vi "enablePWM.vi"(0 "MotorControllerClass in":refnum<class "MotorControllerClass.lvclass">, 3 "error in (no error)":errorcluster) -> (7 "MotorControllerClass out":refnum<class "MotorControllerClass.lvclass">, 10 "error out":errorcluster)   [LabVIEW 2018, in "MotorControllerClass.lvclass"]
uses:
  BMS/MotorControllerClass.lvclass
  <vilib>/CANopenLib/CANOPEN.llb/CANopen Convert To Data [U16].vi
  <vilib>/CANopenLib/CANOPEN.llb/CANopen Convert To Data [I32].vi
  <vilib>/CANopenLib/CANOPEN.llb/CANopen Convert To Data [I16].vi
panel:
  in  "targetVelocity":i32
  in  "targetTorque":i16
  out "interface object out":refnum<k20>
  in  "interface object in":refnum<k20>
  in  "CANopen data in":u8[](array[numeric])=[0, 0, 0, 0, 0, 0, 0, 0] format="%.0x"
  in  "PDOChannel":u8(ring) items=["PDO 1", "PDO 2", "PDO 3", "PDO 4"]
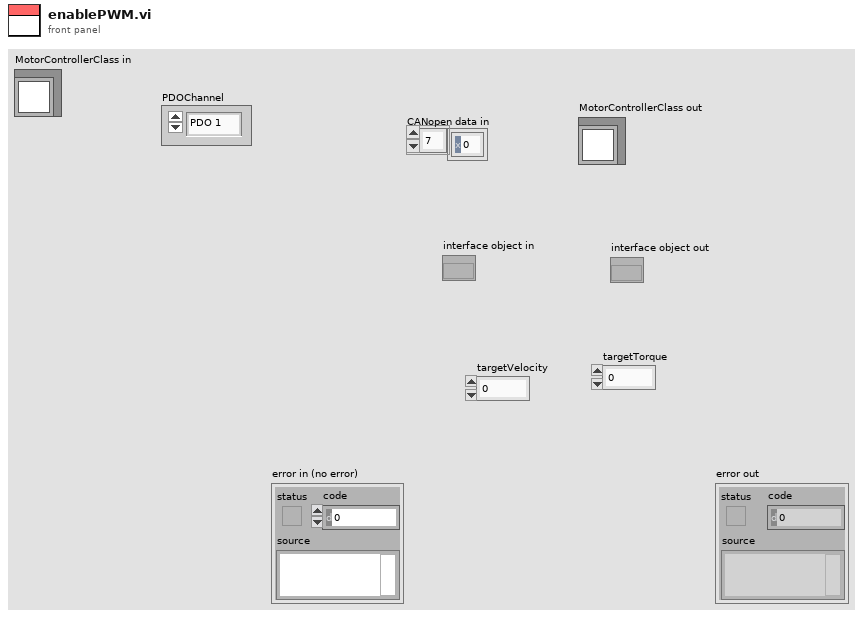
[diagram p1: front panel]
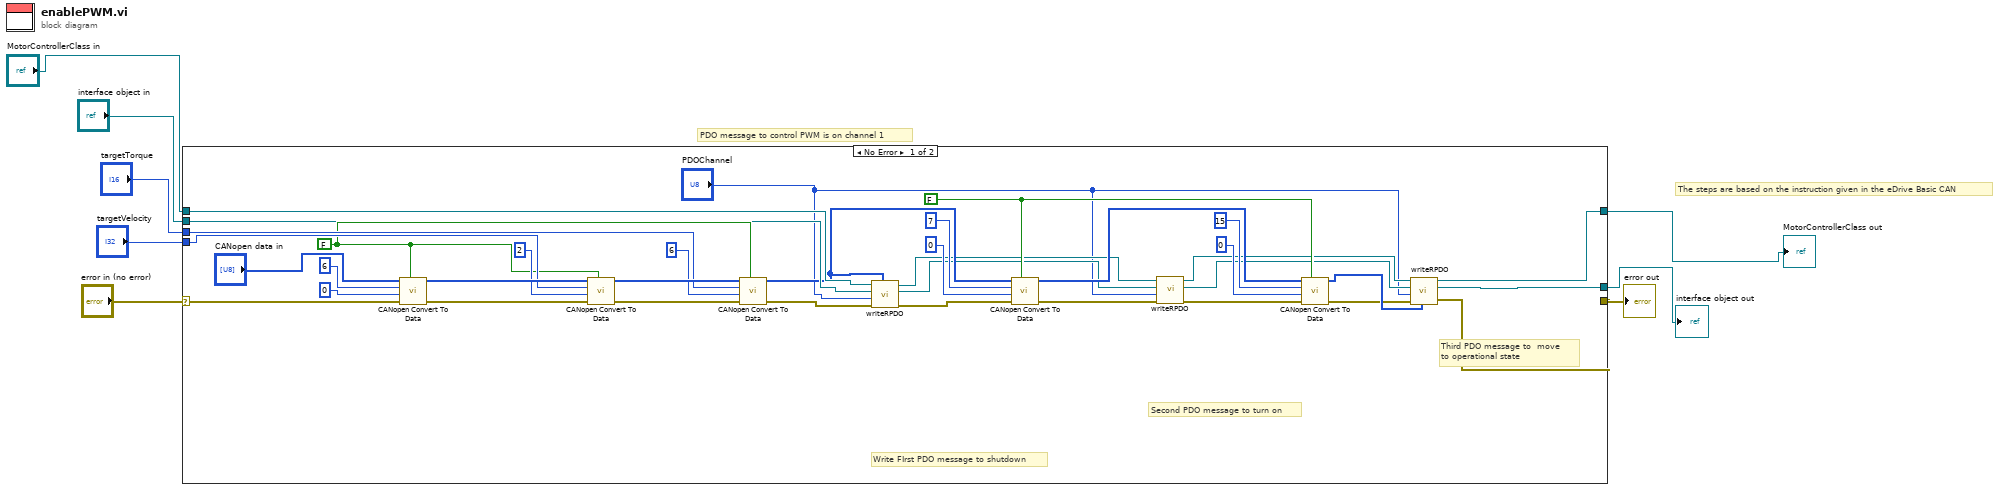
[diagram p0: block diagram]
diagram:
  # "The steps are based on the instruction given in the eDrive Basic CAN"
  # "PDO message to control PWM is on channel 1"
  n1 = case shown="No Error" "error in (no error)" {
    selector: "error in (no error)" -> [w42 w47]
    tunnel: [w9 w47] -> w7
    tunnel: [w11 w46] -> w1
    tunnel: "MotorControllerClass in" -> [w25 w46]
    tunnel: "interface object in" -> [w24 w45]
    tunnel: "targetTorque" -> [w34 _]
    tunnel: "targetVelocity" -> [w38 _]
    tunnel: [w10 w45] -> w3
    frame No Error {
      w28 = FALSE ("trim")
      w32 = FALSE ("trim")
      # "Third PDO message to  move \nto operational state"
      # "Second PDO message to turn on"
      # "Write FIrst PDO message to shutdown"
      n2 = call-poly <vilib>:"CANopen Convert To Data.vi"("trim"=w32, "error in (no error)"=w42, "offset (0)"=u32 0, "unsigned 16-bit integer"=u16 6 ("element"), "CANopen data in"="CANopen data in") -> ("error out"=w40:errorcluster, "CANopen data out"=w39:u8[])  [unwired: 5 in]
      n3 = call-poly <vilib>:"CANopen Convert To Data.vi"("trim"=w32, "error in (no error)"=w40, "offset (0)"=u32 2, "signed 32-bit integer"=w38, "CANopen data in"=w39) -> ("error out"=w36:errorcluster, "CANopen data out"=w35:u8[])  [unwired: 5 in]
      n4 = call-poly <vilib>:"CANopen Convert To Data.vi"("trim"=w32, "error in (no error)"=w36, "offset (0)"=u32 6, "signed 16-bit integer"=w34, "CANopen data in"=w35) -> ("error out"=w23:errorcluster, "CANopen data out"=w22:u8[])  [unwired: 5 in]
      n5 = call "writeRPDO.vi"("RPDO data"=w22, "error in (no error)"=w23, "PDOChannel"="PDOChannel", "interface object in"=w24, "MotorControllerClass in"=w25) -> ("error out"=w21:errorcluster, "interface object out"=w19:refnum<k20>, "MotorControllerClass out"=w20:refnum<class "MotorControllerClass.lvclass">)  [unwired: 4 in]
      n6 = call-poly <vilib>:"CANopen Convert To Data.vi"("trim"=w28, "error in (no error)"=w21, "offset (0)"=u32 0, "unsigned 16-bit integer"=u16 7 ("element"), "CANopen data in"=w22) -> ("error out"=w18:errorcluster, "CANopen data out"=w26:u8[])  [unwired: 5 in]
      n7 = call "writeRPDO.vi"("error in (no error)"=w18, "PDOChannel"="PDOChannel", "interface object in"=w19, "MotorControllerClass in"=w20) -> ("error out"=w17:errorcluster, "interface object out"=w14:refnum<k20>, "MotorControllerClass out"=w15:refnum<class "MotorControllerClass.lvclass">)  [unwired: 5 in]
      n8 = call-poly <vilib>:"CANopen Convert To Data.vi"("trim"=w28, "error in (no error)"=w17, "offset (0)"=u32 0, "unsigned 16-bit integer"=u16 15 ("element"), "CANopen data in"=w26) -> ("error out"=w12:errorcluster, "CANopen data out"=w16:u8[])  [unwired: 5 in]
      n9 = call "writeRPDO.vi"("RPDO data"=w16, "error in (no error)"=w12, "PDOChannel"="PDOChannel", "interface object in"=w14, "MotorControllerClass in"=w15) -> ("error out"=w9:errorcluster, "interface object out"=w10:refnum<k20>, "MotorControllerClass out"=w11:refnum<class "MotorControllerClass.lvclass">)  [unwired: 4 in]
    }
    frame Error {
    }
  }
  "error out" <- w7
  "interface object out" <- w3
  "MotorControllerClass out" <- w1
